vi "HostEventNodeTest.vi"() -> ()   [LabVIEW 2014]
panel:
  in  "OK Button":bool
  out "Loop1":i32
  out "Loop2":i32
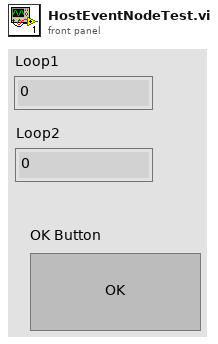
[diagram p1: front panel]
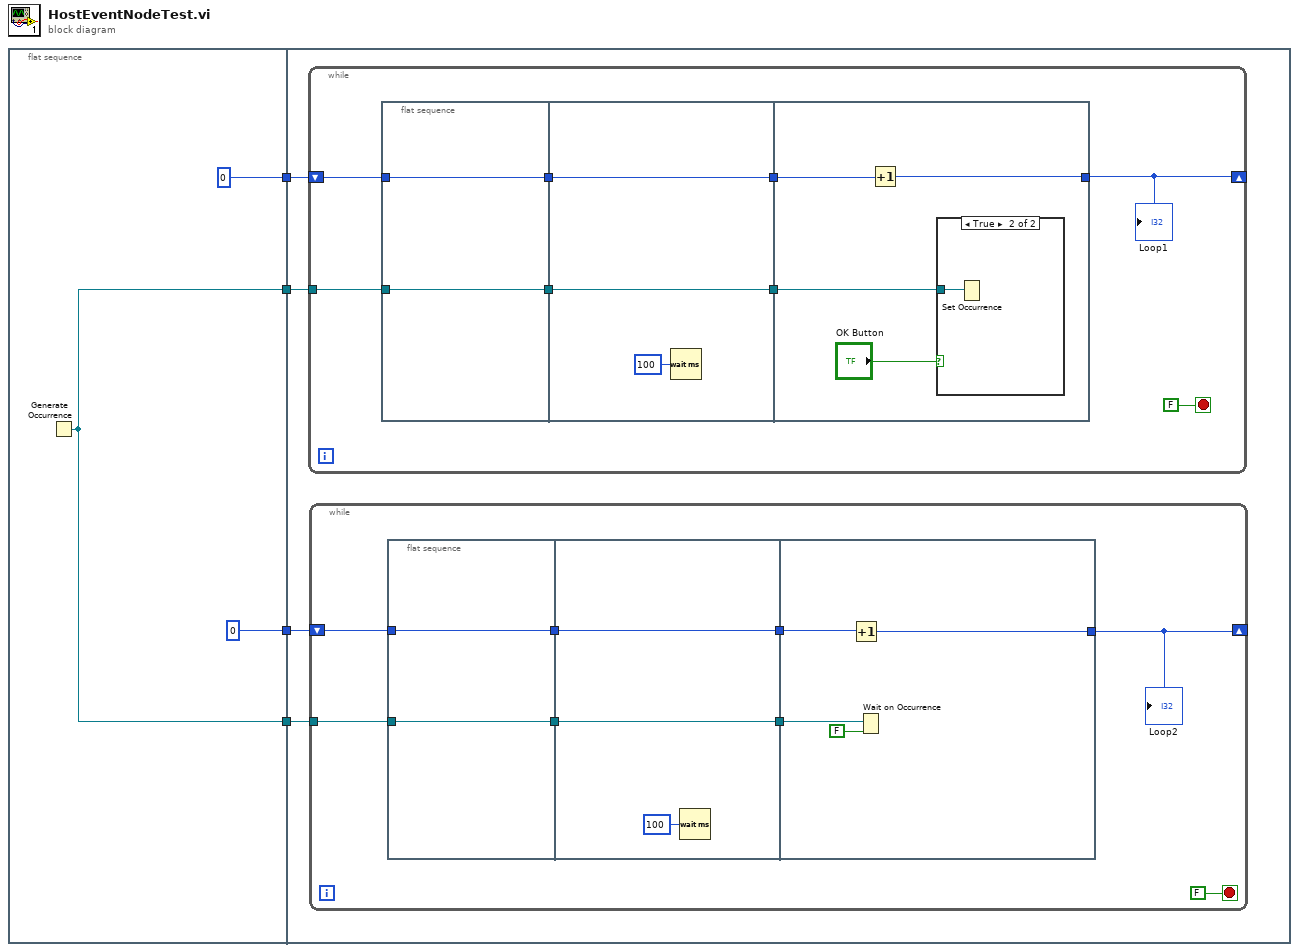
[diagram p0: block diagram]
diagram:
  n1 = flat-sequence {
    tunnel: [0] -> w4
    tunnel: [0] -> w3
    tunnel: [w5] -> w2
    tunnel: [w5] -> w1
    tunnel: w4 -> [w11]
    tunnel: w3 -> [w10]
    tunnel: w2 -> [w9]
    tunnel: w1 -> [w8]
    frame #0 {
      n2 = Generate Occurrence() -> (w5:refnum<k4>)
    }
    frame #1 {
      n3 = while {
        shift-right: [w35] -> _
        shift-left: w10 -> [w32]
        tunnel: w8 -> [w29]
        stop <- FALSE stop-if-true
        n4 = flat-sequence {
          tunnel: [w38] -> w33
          tunnel: w32 -> [w38]
          tunnel: [w37] -> w30
          tunnel: w29 -> [w37]
          tunnel: [w40] -> w34
          tunnel: w33 -> [w40]
          tunnel: [w39] -> w31
          tunnel: w30 -> [w39]
          tunnel: [w44] -> w35
          tunnel: w34 -> [w45]
          tunnel: w31 -> [w42]
          frame #0 {
          }
          frame #1 {
            n5 = Wait (ms)(milliseconds to wait=u32 100) -> ()  [unwired: 1 out]
          }
          frame #2 {
            n6 = Increment(x=w45) -> (x+1=w44:i32)
            n7 = case shown="True" "OK Button" {
              tunnel: w42 -> [_ w46]
              frame False {
              }
              frame True {
                n8 = Set Occurrence(w46) -> ()
              }
            }
          }
        }
        "Loop1" <- w35
      }
      n9 = while {
        shift-right: [w13] -> _
        shift-left: w11 -> [w15]
        tunnel: w9 -> [w12]
        stop <- FALSE stop-if-true
        n10 = flat-sequence {
          tunnel: [w20] -> w17
          tunnel: [w21] -> w16
          tunnel: w15 -> [w21]
          tunnel: w12 -> [w20]
          tunnel: [w23] -> w18
          tunnel: w17 -> [w23]
          tunnel: w16 -> [w22]
          tunnel: [w22] -> w14
          tunnel: w18 -> [w28]
          tunnel: w14 -> [w27]
          tunnel: [w26] -> w13
          frame #0 {
          }
          frame #1 {
            n11 = Wait (ms)(milliseconds to wait=u32 100) -> ()  [unwired: 1 out]
          }
          frame #2 {
            n12 = Increment(x=w27) -> (x+1=w26:i32)
            n13 = Wait on Occurrence(1:FALSE ("ignore previous (T)"), 2:w28) -> ()  [unwired: 1 in, 1 out]
          }
        }
        "Loop2" <- w13
      }
    }
  }
